vi "closed_loop.vi"() -> ()   [LabVIEW 2020]
uses:
  <vilib>/addons/control/pid/NI_PID_autopid.lvlib
panel:
  out "Waveform Chart 2":cluster{"SetPoint":dbl, dbl}(graph)={"SetPoint"=80.0, 78.8394302225639}
  out "Waveform Chart":cluster{dbl, dbl}(graph)={70.49572659929031, 71.71717171717172}
  in  "Alarma Nivel Bajo?":dbl=20.0
  in  "Alarma Nivel Alto?":dbl=85.0
  out "N. Bajo":bool
  out "N. Alto":bool
  out "Entrada":bool=TRUE
  out "% Caudal Ent":dbl=71.71717171717172 format="%#_4g"
  out "% Apertura Valvula":dbl=70.49572659929031 format="%#_4g"
  in  "H inicial Simulación":dbl=25.0
  out "Altura":dbl=78.8394302225639 format="%#_3g"
  out "Valvula":bool=TRUE
  in  "stop":bool
  in  "Caudal de Entrada":dbl(slide)=0.7171717171717172 scale=0.0..1.0
  out "Tanque":dbl(slide)=25.080385852090032 scale=0.0..100.0
  in  "Parámetros PID":T1={"SetPoint"=80.0, "P Gain"=3.0, "I time"=0.08, "D time"=0.0}
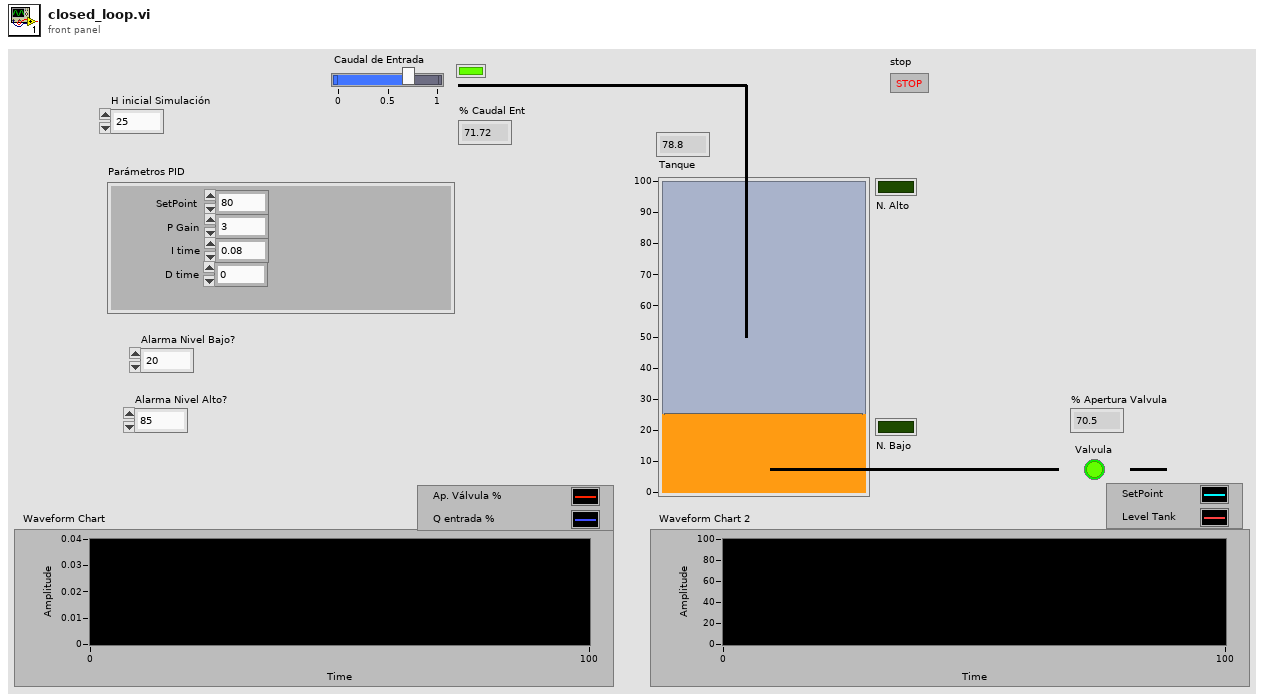
[diagram p1: front panel]
types:
  T1 = cluster{"SetPoint":dbl, "P Gain":dbl, "I time":dbl, "D time":dbl}
  T2 = cluster{"P Gain":dbl, "I time":dbl, "D time":dbl}
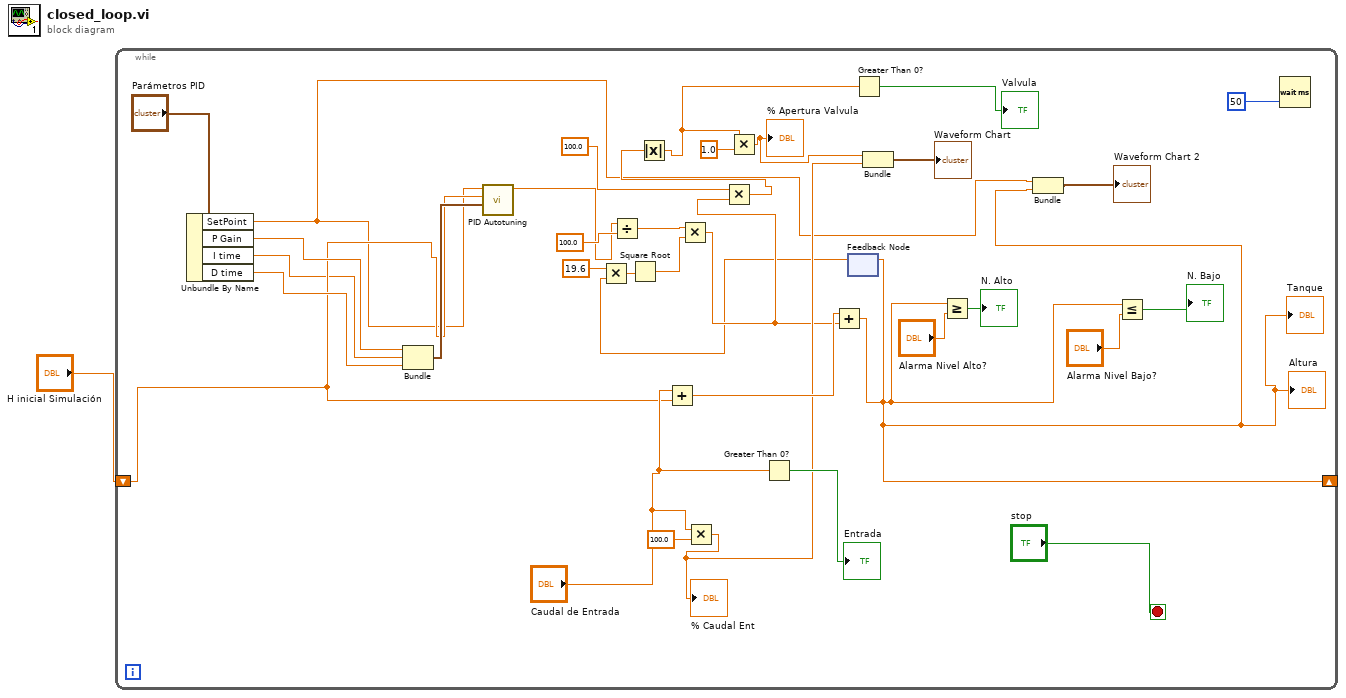
[diagram p0: block diagram]
diagram:
  n1 = while {
    shift-right: [w10] -> _
    shift-left: "H inicial Simulación" -> [w4]
    stop <- "stop" stop-if-true
    n2 = Unbundle By Name("Parámetros PID") -> ("SetPoint"=w3:dbl, "P Gain"=w7:dbl, "I time"=w2:dbl, "D time"=w6:dbl)
    n3 = Bundle("P Gain"=w7, "I time"=w2, "D time"=w6) -> (w5:T2)  [unwired: 1 in]
    n4 = call <vilib>:"PID Autotuning.vi"("PID gains"=w5, "process variable"=w4, "setpoint"=w3) -> ("output"=w8:dbl)  [unwired: 5 in, 3 out]
    n5 = Divide(x=w8, y=100.0) -> (x/y=w17:dbl)
    n6 = Add(x="Caudal de Entrada", y=w4) -> (x+y=w33:dbl)
    n7 = Multiply(x="Caudal de Entrada", y=100.0) -> (x*y=w19:dbl)
    "% Caudal Ent" <- w19
    n8 = Greater Than 0?(x="Caudal de Entrada") -> (x > 0?=→"Entrada":bool)
    n9 = feedback #1() -> (w9:dbl)  [unwired: 1 in]
    n10 = Multiply(x=19.6, y=w9) -> (x*y=w16:dbl)
    n11 = Square Root(x=w16) -> (sqrt(x)=w14:dbl)
    n12 = Multiply(x=w17, y=w14) -> (x*y=w13:dbl)
    n13 = Multiply(x=100.0, y=w13) -> (x*y=w11:dbl)
    n14 = Absolute Value(x=w11) -> (abs(x)=w25:dbl)
    n15 = Multiply(x=w25, y=1.0) -> (x*y=w20:dbl)
    "% Apertura Valvula" <- w20
    n16 = Add(x=w33, y=w13) -> (x+y=w10:dbl)
    "Tanque" <- w10
    "Altura" <- w10
    n17 = feedback-in #1(w10) -> ()
    n18 = Greater Than 0?(x=w25) -> (x > 0?=→"Valvula":bool)
    n19 = Bundle(w20, w19) -> (→"Waveform Chart":cluster{dbl, dbl})  [unwired: 1 in]
    n20 = Greater Or Equal?(x=w10, y="Alarma Nivel Alto?") -> (x >= y?=→"N. Alto":bool)
    n21 = Bundle("SetPoint"=w3, w10) -> (→"Waveform Chart 2":cluster{"SetPoint":dbl, dbl})  [unwired: 1 in]
    n22 = Less Or Equal?(x=w10, y="Alarma Nivel Bajo?") -> (x <= y?=→"N. Bajo":bool)
    n23 = Wait (ms)(milliseconds to wait=50) -> ()  [unwired: 1 out]
  }
